vi "quaternion to euler angles.vi"(2 "Degrees? (true)":bool=TRUE, 3 "Quaternion":dbl[](array[numeric])=[1.0, 0.0, 0.0, 0.0]) -> (1 "Euler angles":dbl[](array[numeric]))   [LabVIEW 2021, in "IMU Display.lvlib"]
uses:
  IMU Display.lvlib
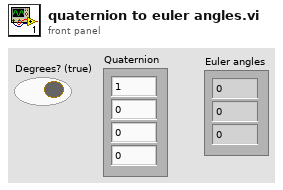
[diagram p1: front panel]
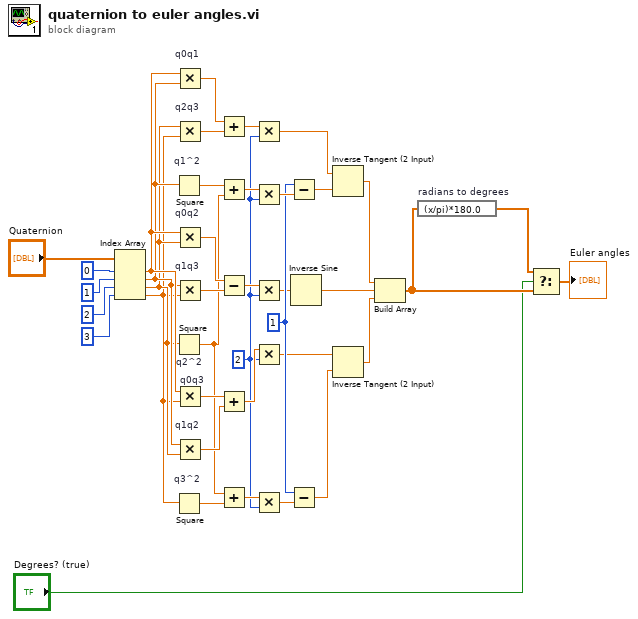
[diagram p0: block diagram]
diagram:
  w13 = 1
  w16 = 2
  n1 = Index Array(array="Quaternion", index #1=0 ("index"), index #2=1 ("index"), index #3=2 ("index"), index #4=3 ("index")) -> (element #1=w30:dbl, element #2=w29:dbl, element #3=w28:dbl, element #4=w27:dbl)
  n2 = Square "q1^2"(x=w29) -> (x^2=w26:dbl)
  n3 = Square "q2^2"(x=w28) -> (x^2=w23:dbl)
  n4 = Square "q3^2"(x=w27) -> (x^2=w22:dbl)
  n5 = Multiply "q0q1"(x=w30, y=w29) -> (x*y=w34:dbl)
  n6 = Multiply "q2q3"(x=w28, y=w27) -> (x*y=w33:dbl)
  n7 = Multiply "q0q2"(x=w30, y=w28) -> (x*y=w32:dbl)
  n8 = Multiply "q1q3"(x=w29, y=w27) -> (x*y=w31:dbl)
  n9 = Multiply "q0q3"(x=w30, y=w27) -> (x*y=w25:dbl)
  n10 = Multiply "q1q2"(x=w29, y=w28) -> (x*y=w24:dbl)
  n11 = Add(x=w34, y=w33) -> (x+y=w21:dbl)
  n12 = Add(x=w26, y=w23) -> (x+y=w20:dbl)
  n13 = Subtract(x=w32, y=w31) -> (x-y=w19:dbl)
  n14 = Add(x=w25, y=w24) -> (x+y=w18:dbl)
  n15 = Add(x=w23, y=w22) -> (x+y=w17:dbl)
  n16 = Multiply(x=w21, y=w16) -> (x*y=w10:dbl)
  n17 = Multiply(x=w20, y=w16) -> (x*y=w15:dbl)
  n18 = Multiply(x=w19, y=w16) -> (x*y=w8:dbl)
  n19 = Multiply(x=w18, y=w16) -> (x*y=w9:dbl)
  n20 = Multiply(x=w17, y=w16) -> (x*y=w14:dbl)
  n21 = Subtract(x=w13, y=w15) -> (x-y=w12:dbl)
  n22 = Subtract(x=w13, y=w14) -> (x-y=w11:dbl)
  n23 = Inverse Sine(1:w8) -> (0:w6:dbl)
  n24 = Inverse Tangent (2 Input)(1:w12, 2:w10) -> (0:w7:dbl)
  n25 = Inverse Tangent (2 Input)(1:w11, 2:w9) -> (0:w5:dbl)
  n26 = Build Array(w7, w6, w5) -> (w3:dbl[])
  n27 = expression code="(x/pi)*180.0" "radians to degrees"(w3) -> (w4:dbl[])
  n28 = Select(t=w4, s="Degrees? (true)", f=w3) -> (s? t:f=→"Euler angles":dbl[])
